vi "WritePacket.vi"(8 "Payload":u8[](array[numeric]), 9 "Type":u8=31, 10 "Status":u8, 11 "Refnum in":refnum<k20>) -> (2 "PacketOut":u8[](array[numeric]))   [LabVIEW 2011]
uses:
  <vilib>/Utility/error.llb/Error Cluster From Error Code.vi
  <vilib>/rvi/errors/niLvFpgaAdjustHostInterfaceError.vi
  <vilib>/rvi/interface/nirviMethod/nirviMethod.xnode
  <vilib>/FPGAPlugInAG/Dynamic/niLvFpga_WriteFifo_Dynamic.vi
  <vilib>/rvi/errors/niLvFpgaMergeErrorWithErrorCode.vi
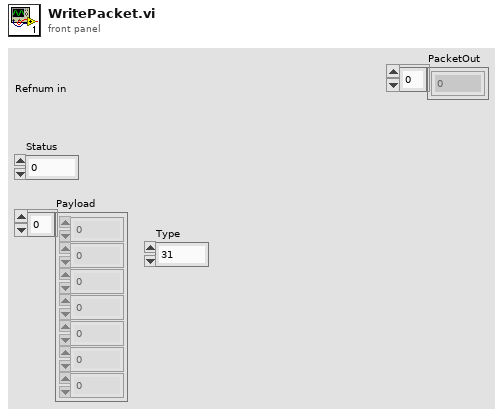
[diagram p1: front panel]
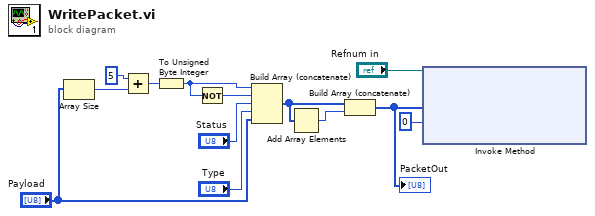
[diagram p0: block diagram]
diagram:
  n1 = Array Size(array="Payload") -> (size(s)=w6:i32)
  n2 = Add(x=5, y=w6) -> (x+y=w8:i32)
  n3 = To Unsigned Byte Integer(number=w8) -> (unsigned 8bit integer=w9:u8)
  n4 = Not(x=w9) -> (.not. x?=w10:u8)
  n5 = Build Array (concatenate)(w9, w10, "Status", "Type", "Payload") -> (w11:u8[])
  n6 = Add Array Elements(numeric array=w11) -> (sum=w12:u8)
  n7 = Build Array (concatenate)(w11, w12) -> (w13:u8[])
  "PacketOut" <- w13
  n8 = xnode "Invoke Method"("FPGA VI Reference In"="Refnum in", "Data"=w13, "Timeout (ms)"=0 ("WriteTimeout")) -> ()  [unwired: 1 in, 3 out]
